vi "Set Property.vi"(10 "Ctl Ref":refnum<vi>, 11 "UIP In":refnum<class "TipStripUIP.lvclass">) -> (0 "Error Out":errorcluster, 3 "UIP Out":refnum<class "TipStripUIP.lvclass">)   [LabVIEW 2020, in "UIM.lvlib" / "TipStripUIP.lvclass"]
doc: "Modify this method to implement functionality for applying the UIP data to the property from VI Server Control."
uses:
  TipStripUIP.lvclass
  TipStripUIP.lvclass/TipStripUIP.ctl
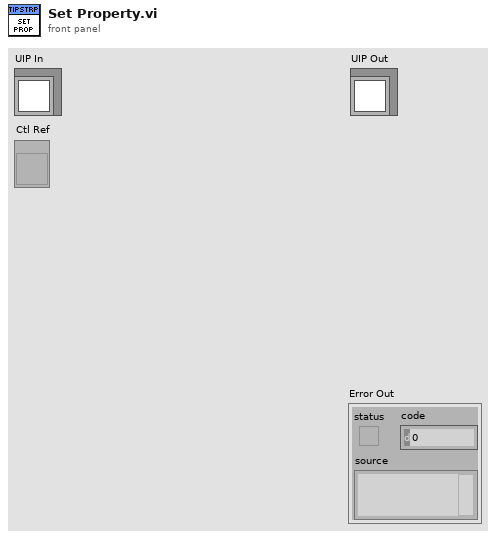
[diagram p1: front panel]
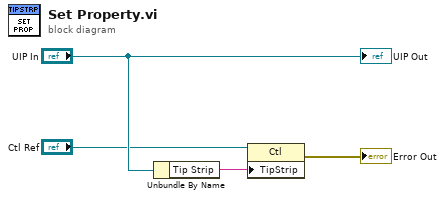
[diagram p0: block diagram]
diagram:
  n1 = Unbundle By Name("UIP In") -> ("Tip Strip"=w2:string)
  n2 = property class="Ctl"(reference="Ctl Ref", "TipStrip"=w2) -> (error out=→"Error Out":errorcluster)  [unwired: 1 in, 1 out]
  "UIP Out" <- "UIP In"
